vi "GUI Panel Control.vi"(7 "action (open panel)":T1, 8 "error in (no error)":errorcluster, 11 "vi path":path) -> (0 "error out":errorcluster)   [LabVIEW 2020]
doc: "Manual control of the VI panel."
uses:
  GUI Panel Control Action.ctl
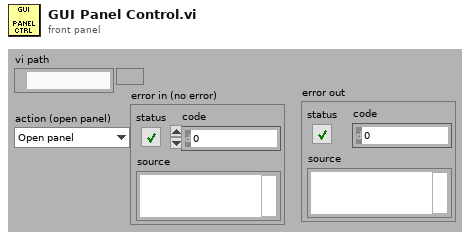
[diagram p1: front panel]
types:
  T1 = typedef "GUI Panel Control Action.ctl" = enum16{"Open panel", "Close panel", "Bring To Front"}
  T2 = enum32{"Invalid", "Standard", "Closed", "Hidden", "Minimized", "Maximized"}
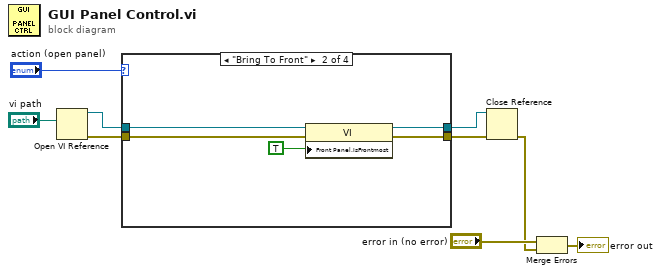
[diagram p0: block diagram]
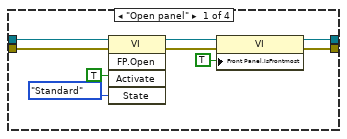
[diagram p2: hidden frame]
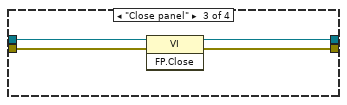
[diagram p3: hidden frame]
diagram:
  n1 = Open VI Reference(vi path="vi path") -> (vi reference=w5:refnum<vi>, error out=w7:errorcluster)  [unwired: 5 in]
  n2 = case shown="\"Bring To Front\"" "action (open panel)" {
    tunnel: [w17 w22 w25 w29] -> w9
    tunnel: [w16 w21 w24 w28] -> w8
    tunnel: w7 -> [w15 w19 w27 w29]
    tunnel: w5 -> [w14 w20 w26 w28]
    frame "Open panel" {
      n3 = invoke class="VI" method="FP.Open"(reference=w14, error in=w15, "Activate"=TRUE ("Activate?"), "State"=T2."Standard") -> (reference out=w12:refnum<vi>, error out=w13:errorcluster)  [unwired: 1 in, 3 out]
      n4 = property class="VI"(reference=w12, error in=w13, "Front Panel.IsFrontmost"=TRUE ("Front Panel Window:Is Frontmost")) -> (reference out=w16:refnum<vi>, error out=w17:errorcluster)
    }
    frame "Bring To Front" {
      n5 = property class="VI"(reference=w20, error in=w19, "Front Panel.IsFrontmost"=TRUE ("Front Panel Window:Is Frontmost")) -> (reference out=w21:refnum<vi>, error out=w22:errorcluster)
    }
    frame "Close panel" {
      n6 = invoke class="VI" method="FP.Close"(reference=w26, error in=w27) -> (reference out=w24:refnum<vi>, error out=w25:errorcluster)  [unwired: 1 in, 1 out]
    }
    frame Default {
    }
  }
  n7 = Close Reference(reference=w8, error in (no error)=w9) -> (error out=w2:errorcluster)
  n8 = Merge Errors("error in (no error)", w2) -> (→"error out":errorcluster)
